vi "Plot subChangeDetector.vi"(10 "value":variant) -> (1 "changed?":bool, 2 "previous value":variant)   [LabVIEW 2020, in "3D Plot.lvclass"]
uses:
  <vilib>/Math Plots/3D Math Plots/3D Plot/3D Plot/3D Plot.lvclass
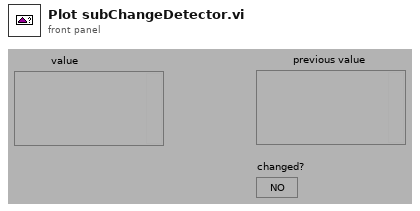
[diagram p1: front panel]
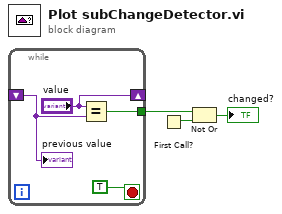
[diagram p0: block diagram]
diagram:
  n1 = while {
    tunnel: [w5] -> w3
    shift-left: _ -> [w7]
    shift-right: ["value"] -> _
    stop <- TRUE stop-if-true
    n2 = Equal?(x="value", y=w7) -> (x = y?=w5:bool)
    "previous value" <- w7
  }
  n3 = First Call?() -> (First Call?: T/F=w2:bool)
  n4 = Not Or(1:w2, 2:w3) -> (0:→"changed?":bool)
